vi "Linear_kernel.vi"(8 "error in":errorcluster caption="entrée d'erreur", 9 "Y":string[][](array[string]), 10 "X":string[][](array[string]), 11 "linear_kernel":cluster{"dense_output":bool}={"dense_output"=TRUE}) -> (0 "error out":errorcluster caption="sortie d'erreur", 3 "Data":T1)   [LabVIEW 2020]
doc: "Compute the linear kernel between X and Y.\n\nParameters : \n\n- X : array of shape (n_samples_1, n_features)\n\n- Y : array of shape (n_samples_2, n_features)\ndense_outputboolean (optional), default True\nWhether to return dense output even when the input is sparse. If False, the output is sparse if both input arrays are sparse.\n\nReturns : \n\n- Gram matrix : array of shape (n_samples_1, n_samples_2)"
uses:
  Linear_kernel.lvclass
panel:
  out "Linear_kernel.lvclass":refnum<class "Linear_kernel.lvclass">
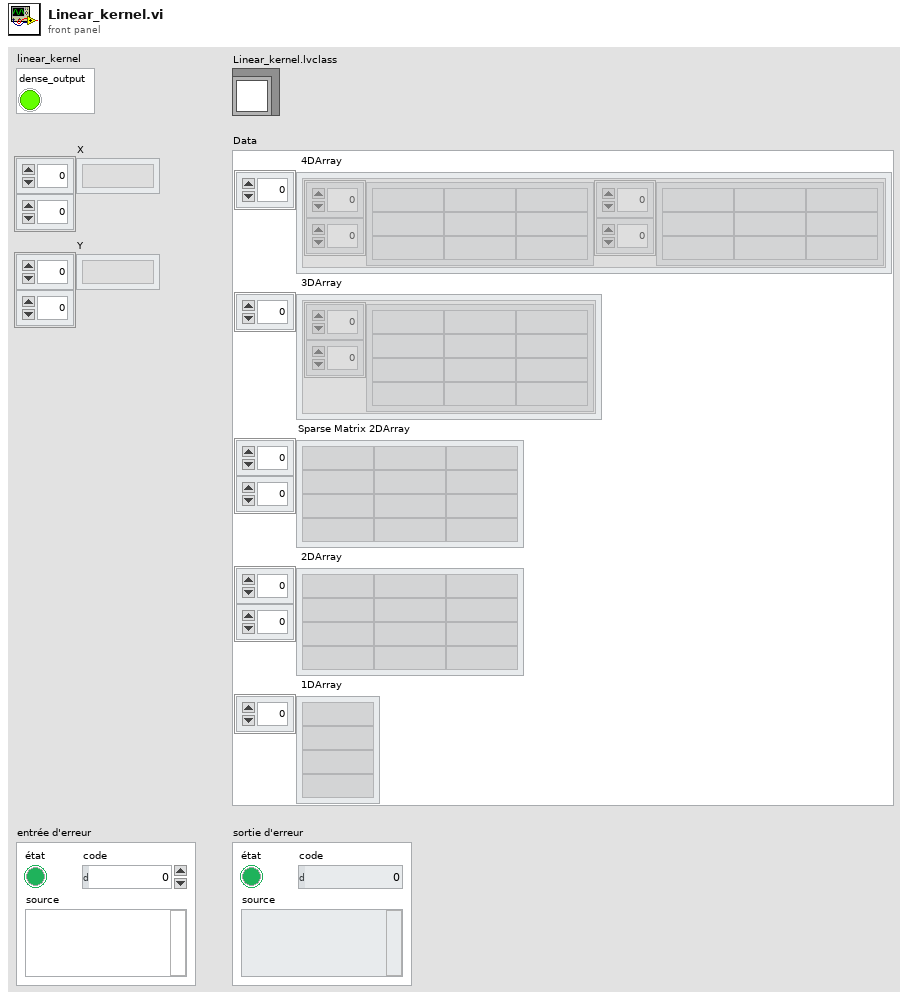
[diagram p1: front panel]
types:
  T1 = cluster{" 4DArray":cluster{"1":string[][], "2":string[][]}[], " 3DArray":cluster{"Tableau":string[][]}[], "Sparse Matrix 2DArray":string[][], " 2DArray":string[][], " 1DArray":string[]}
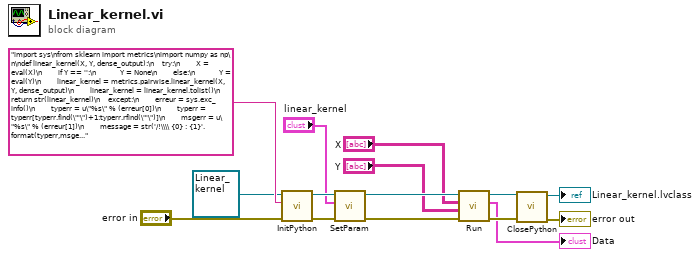
[diagram p0: block diagram]
diagram:
  n1 = call-dynamic "InitPython.vi"("error in (no error)"="error in", "Python Instruction"="import sys\nfrom sklearn import metrics\nimport numpy as np\n\ndef linear_kernel(X, Y, dense_output):\n    try:\n        X = eval(X)\n        if Y == '':\n            Y = None\n        else:\n            Y = eval(Y)\n        linear_kernel = metrics.pairwise.linear_kernel(X, Y, dense_output)\n        linear_kernel = linear_kernel.tolist()\n        return str(linear_kernel)\n    except:\n        erreur = sys.exc_info()\n        typerr = u\"%s\" % (erreur[0])\n        typerr = typerr[typerr.find(\"'\")+1:typerr.rfind(\"'\")]\n        msgerr = u\"%s\" % (erreur[1])\n        message = str('/!\\\\ {0} : {1}'. format(typerr,msgerr))\n        return message", "Scikit-learn en entrée"=refnum<class "Linear_kernel.lvclass"> refnum ("Linear_kernel.lvclass")) -> ("error out"=w12:errorcluster, "Scikit-learn en sortie"=w11:refnum<class "Linear_kernel.lvclass">)  [unwired: 7 in]
  n2 = call-dynamic "SetParam.vi"("error in (no error)"=w12, "linear_kernel"="linear_kernel", "Linear_kernel.lvclass"=w11) -> ("error out"=w9:errorcluster, "Linear_kernel.lvclass"=w8:refnum<class "Linear_kernel.lvclass">)  [unwired: 7 in]
  n3 = call-dynamic "Run.vi"("error in (no error)"=w9, "Y"="Y", "X"="X", "Linear_kernel.lvclass"=w8) -> ("error out"=w6:errorcluster, "Data"=→"Data":T1, "Linear_kernel.lvclass"=w7:refnum<class "Linear_kernel.lvclass">)  [unwired: 5 in]
  n4 = call-dynamic "ClosePython.vi"("error in (no error)"=w6, "Scikit-learn en entrée"=w7) -> ("error out"=→"error out":errorcluster, "Scikit-learn en sortie"=→"Linear_kernel.lvclass":refnum<class "Linear_kernel.lvclass">)  [unwired: 8 in]
